vi "Correct Data.vi"(8 "error in (no error)":errorcluster, 10 "Data In":refnum<class "Data.lvclass">, 11 "Vaisala in":refnum<class "Vaisala.lvclass">) -> (0 "error out":errorcluster, 2 "Data Out":refnum<class "Data.lvclass">, 3 "Vaisala out":refnum<class "Vaisala.lvclass">)   [LabVIEW 2015, in "Vaisala Library.lvlib" / "Vaisala.lvclass"]
uses:
  Vaisala.lvclass
  <vilib>/gmath/NI_Gmath.lvlib
  Data/Vaisala Data.lvclass
  <vilib>/MSR Consulting, LLC/General Reuse/Data/Data.lvclass
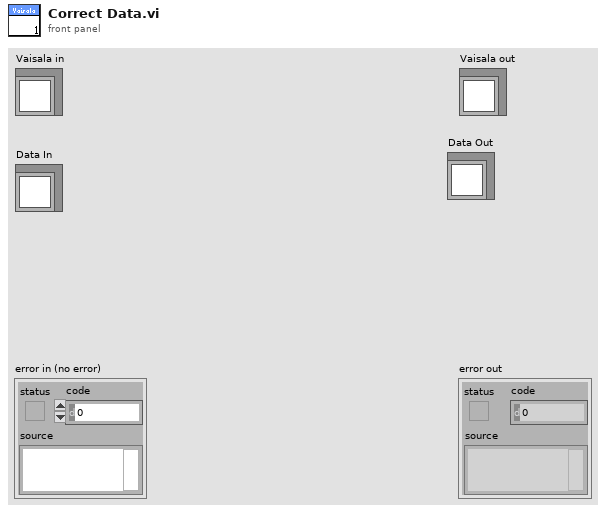
[diagram p1: front panel]
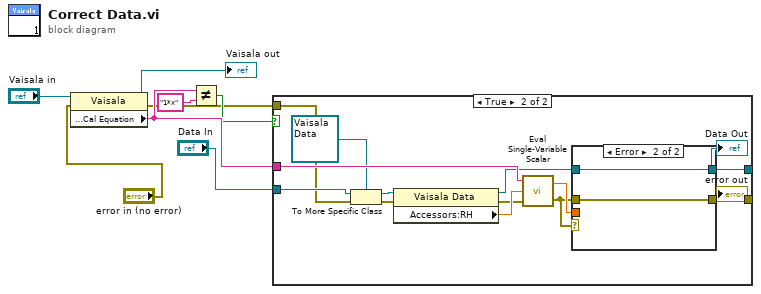
[diagram p0: block diagram]
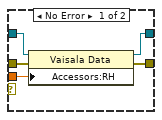
[diagram p3: hidden frame]
diagram:
  n1 = property class="Vaisala"(reference="Vaisala in", error in="error in (no error)") -> (reference out=→"Vaisala out":refnum<class "Vaisala.lvclass">, error out=w1:errorcluster, "Accessors:Cal Equation"=w9:string)
  n2 = Not Equal?(x=w9, y="1*x") -> (x != y?=w7:bool)
  n3 = case shown="True" w7 {
    tunnel: w9 -> [_ w25]
    tunnel: "Data In" -> [w12 w24]
    tunnel: [w12 w18] -> w5
    tunnel: w1 -> [w11 w14]
    tunnel: [w11 w13] -> w4
    frame False {
    }
    frame True {
      n4 = To More Specific Class(target class=refnum<class "Vaisala Data.lvclass"> refnum ("Vaisala Library.lvlib:Vaisala Data"), reference=w24, error in=w14) -> (specific class reference=w22:refnum<class "Vaisala Data.lvclass">, error out=w15:errorcluster)
      n5 = property class="Vaisala Data"(reference=w22, error in=w15) -> (reference out=w19:refnum<class "Vaisala Data.lvclass">, error out=w16:errorcluster, "Accessors:RH"=w21:dbl)
      n6 = call <vilib>:"Eval Single-Variable Scalar.vi"("error in (no error)"=w16, "x value"=w21, "formula"=w25) -> ("error out"=w17:errorcluster, "y value"=w20:dbl)
      n7 = case shown="Error" w17 {
        tunnel: w20 -> [w30 _]
        tunnel: w17 -> [w29 w31]
        tunnel: w19 -> [w28 w32]
        tunnel: [w27 w32] -> w18
        tunnel: [w26 w31] -> w13
        frame No Error {
          n8 = property class="Vaisala Data"(reference=w28, error in=w29, "Accessors:RH"=w30) -> (reference out=w27:refnum<class "Vaisala Data.lvclass">, error out=w26:errorcluster)
        }
        frame Error {
        }
      }
    }
  }
  "error out" <- w4
  "Data Out" <- w5
